vi "Read PythonVersion.vi"(8 "error in (no error)":errorcluster, 11 "PythonSession in":refnum<class "PythonSession.lvclass">) -> (0 "error out":errorcluster, 2 "PythonVersion":string, 3 "PythonSession out":refnum<class "PythonSession.lvclass">)   [LabVIEW 2022 SP3, in "PythonWrapper.lvlib" / "PythonSession.lvclass"]
uses:
  PythonSession.lvclass
  PythonSession.lvclass/PythonSession.ctl
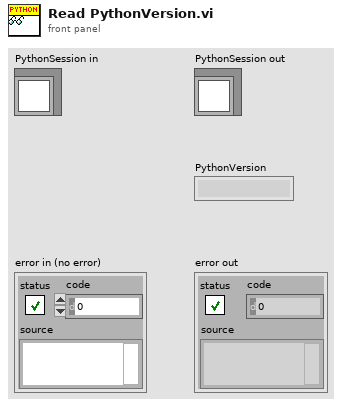
[diagram p1: front panel]
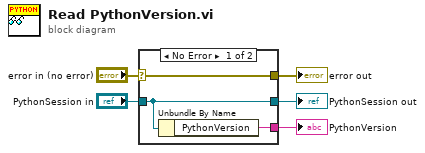
[diagram p0: block diagram]
diagram:
  n1 = case shown="No Error" "error in (no error)" {
    selector: "error in (no error)" -> [w8 w9]
    tunnel: [w8 w9] -> w4
    tunnel: [w7 w10] -> w2
    tunnel: "PythonSession in" -> [w7 w10]
    tunnel: [w6 _] -> w1
    frame No Error {
      n2 = Unbundle By Name(w7) -> ("PythonVersion"=w6:string)
    }
    frame Error {
    }
  }
  "error out" <- w4
  "PythonSession out" <- w2
  "PythonVersion" <- w1
